vi "Configure Math.vi"(0 "VISA resource name":refnum<visa-resource-name>, 1 "Operation (0:None)":i32(ring) items=["None", "Min/Max", "Null", "dB", "dBm", "Limit"], 5 "Null Offset (0)":dbl format="%#_3g", 7 "dB Reference Point (0 dB)":dbl format="%#_3g", 9 "dBm Resistance (600 Ohms)":i32(ring)=600 items=["2"=2, "4"=4, "8"=8, "16"=16, "50"=50, "75"=75, "93"=93, "110"=110, "124"=124, "125"=125, "135"=135, "150"=150, "250"=250, "300"=300, "500"=500, "600"=600, "800"=800, "900"=900, "1000"=1000, "1200"=1200, "8000"=8000], 11 "error in (no error)":errorcluster, 12 "Upper Limit (0)":dbl format="%#_3g", 13 "Lower Limit (0)":dbl format="%#_3g") -> (4 "VISA resource name out":refnum<visa-resource-name>, 15 "error out":errorcluster)   [LabVIEW 2020, in "Agilent 34405.lvlib"]
doc: "Configures the math functions available on the instrument."
uses:
  <instrlib>/Agilent 34405/Agilent 34405.lvlib
panel:
  # "Null Function"
  # "DB Measurements"
  # "Limit"
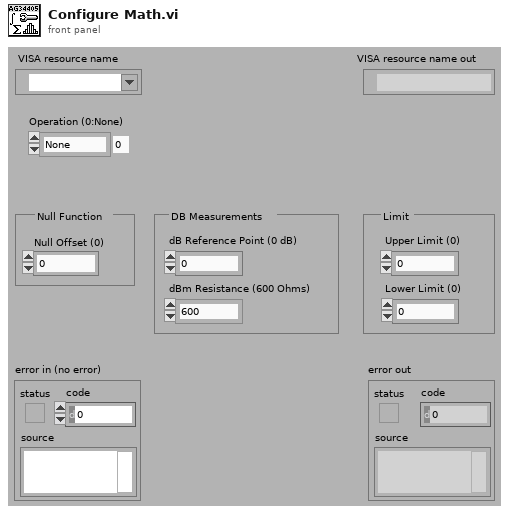
[diagram p1: front panel]
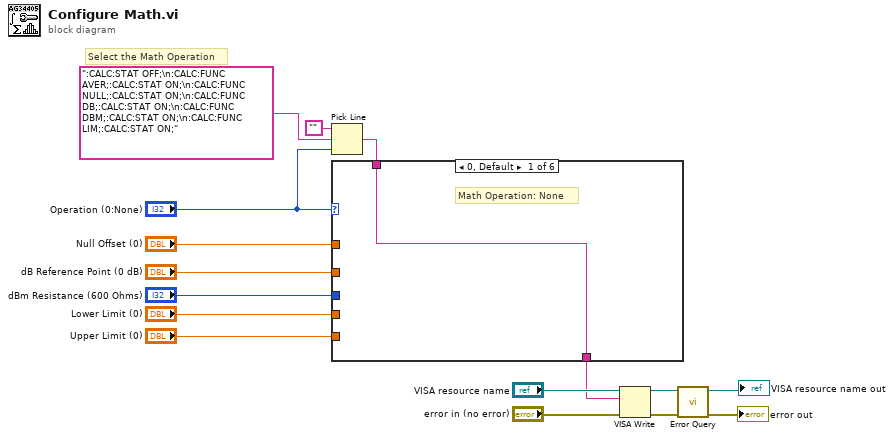
[diagram p0: block diagram]
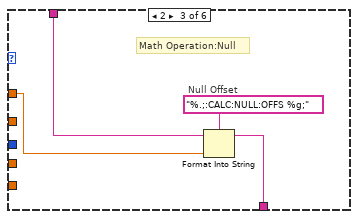
[diagram p3: hidden frame]
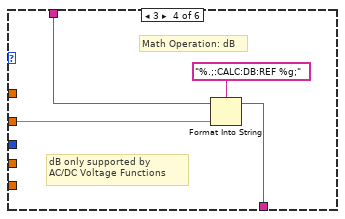
[diagram p4: hidden frame]
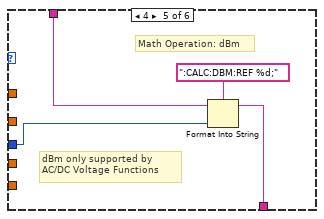
[diagram p5: hidden frame]
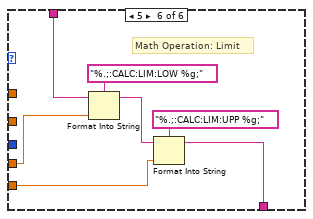
[diagram p6: hidden frame]
diagram:
  # "Select the Math Operation"
  n1 = Pick Line(string ("")="" ("Empty String Constant"), multi-line string=":CALC:STAT OFF;\n:CALC:FUNC AVER;:CALC:STAT ON;\n:CALC:FUNC NULL;:CALC:STAT ON;\n:CALC:FUNC DB;:CALC:STAT ON;\n:CALC:FUNC DBM;:CALC:STAT ON;\n:CALC:FUNC LIM;:CALC:STAT ON;", line index="Operation (0:None)") -> (output string=w15:string)
  n2 = case shown="0, Default" "Operation (0:None)" {
    tunnel: w15 -> [w17 w18 w22 w26 w28 w37]
    tunnel: [w17 w18 w21 w24 w30 w33] -> w6
    tunnel: "Null Offset (0)" -> [_ _ w19 _ _ _]
    tunnel: "dB Reference Point (0 dB)" -> [_ _ _ w23 _ _]
    tunnel: "dBm Resistance (600 Ohms)" -> [_ _ _ _ w27 _]
    tunnel: "Upper Limit (0)" -> [_ _ _ _ _ w32]
    tunnel: "Lower Limit (0)" -> [_ _ _ _ _ w31]
    frame 0, Default {
      # "Math Operation: None"
    }
    frame 1 {
      # "Math Operation: Min/Max"
    }
    frame 2 {
      # "Math Operation:Null"
      # "Null Offset"
      n3 = Format Into String(format string="%.;:CALC:NULL:OFFS %g;", initial string=w22, w19) -> (resulting string=w21:string)  [unwired: 1 in, 1 out]
    }
    frame 3 {
      # "Math Operation: dB"
      # "dB only supported by \nAC/DC Voltage Functions"
      n4 = Format Into String(format string="%.;:CALC:DB:REF %g;", initial string=w26, w23) -> (resulting string=w24:string)  [unwired: 1 in, 1 out]
    }
    frame 4 {
      # "Math Operation: dBm"
      # "dBm only supported by \nAC/DC Voltage Functions"
      n5 = Format Into String(format string=":CALC:DBM:REF %d;", initial string=w28, w27) -> (resulting string=w30:string)  [unwired: 1 in, 1 out]
    }
    frame 5 {
      # "Math Operation: Limit"
      n6 = Format Into String(format string="%.;:CALC:LIM:LOW %g;", initial string=w37, w31) -> (resulting string=w34:string)  [unwired: 1 in, 1 out]
      n7 = Format Into String(format string="%.;:CALC:LIM:UPP %g;", initial string=w34, w32) -> (resulting string=w33:string)  [unwired: 1 in, 1 out]
    }
  }
  n8 = VISA Write(VISA resource name="VISA resource name", write buffer=w6, error in (no error)="error in (no error)") -> (VISA resource name out=w12:refnum<visa-resource-name>, error out=w13:errorcluster)  [unwired: 1 out]
  n9 = call <instrlib>:"Error Query.vi"("error in (no error)"=w13, "VISA resource name"=w12) -> ("error out"=→"error out":errorcluster, "VISA resource name out"=→"VISA resource name out":refnum<visa-resource-name>)  [unwired: 8 out]
